vi "Create User Event.vi"(8 "error in (no error)":errorcluster caption="エラー入力（エラーなし）") -> (0 "error out":errorcluster caption="エラー出力", 3 "User Event":refnum<user-event>, 5 "Event Registration Refnum":refnum<event-registration>)   [LabVIEW 2014]
doc: "ユーザイベントを作成します。"
uses:
  Ctl/Event Cluster.ctl
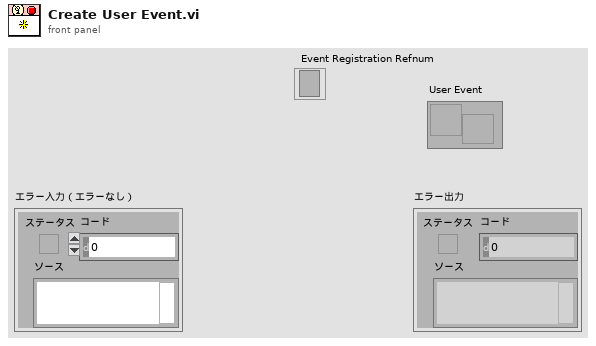
[diagram p1: front panel]
types:
  T1 = typedef "Event Cluster.ctl" = cluster{"コマンド":string, "バリアント":variant}
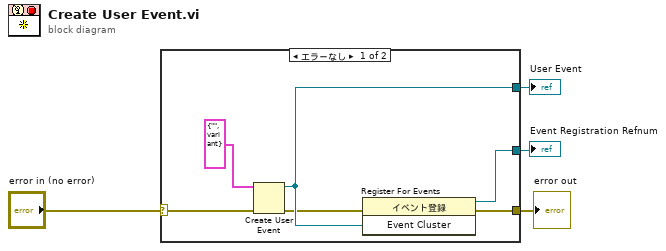
[diagram p0: block diagram]
diagram:
  n1 = case shown="エラーなし" "error in (no error)" {
    selector: "error in (no error)" -> [w6 w11]
    tunnel: [w10 _] -> w2
    tunnel: [w9 _] -> w1
    tunnel: [w7 w11] -> w4
    frame No Error {
      n2 = Create User Event(user event datatype=T1 {"コマンド"="", "バリアント"=variant} ("Event Cluster"), error in=w6) -> (user event=w10:refnum<user-event>, error out=w8:errorcluster)
      n3 = register-events(error in=w8, w10) -> (reference out=w9:refnum<event-registration>, error out=w7:errorcluster)  [unwired: 1 in]
    }
    frame Error {
    }
  }
  "error out" <- w4
  "User Event" <- w2
  "Event Registration Refnum" <- w1
